vi "SetupAOTF.vi"() -> ()   [LabVIEW 2009]
uses:
  AOTFSettings.ctt
panel:
  in  "AOTF Setting":T1={"Laser 1 Output Channel"="5", "AOTF  1 Output Voltage"=5.0, "Laser 2 Output Channel"="6", "AOTF  2 Output Voltage"=5.0, "Laser 3 Output Channel"="1", "AOTF  3 Output Voltage"=0.0, "Pixel per Cycle"=3, "Time per Cycle  / ms"=0.1, "Laser 4 Output Channel"="1", "AOTF  4 Output Voltage"=0.0} {"AOTF  4 Output Voltage" format="%.2f"; "Time per Cycle  / ms" format="%#.3f"; "AOTF  3 Output Voltage" min=0.0 max=10.0 format="%.2f"; "AOTF  2 Output Voltage" min=0.0 max=10.0 format="%.2f"; "AOTF  1 Output Voltage" min=0.0 max=10.0 format="%.2f"}
  in  "Analog Setup":bool
  in  "OK Button":bool
  in  "Cancel Button":bool
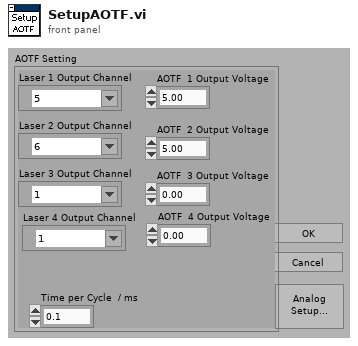
[diagram p1: front panel]
types:
  T1 = typedef "AOTFSettings.ctt" = cluster{"Laser 1 Output Channel":tag, "AOTF  1 Output Voltage":dbl, "Laser 2 Output Channel":tag, "AOTF  2 Output Voltage":dbl, "Laser 3 Output Channel":tag, "AOTF  3 Output Voltage":dbl, "Pixel per Cycle":u16, "Time per Cycle  / ms":dbl, "Laser 4 Output Channel":tag, "AOTF  4 Output Voltage":dbl}
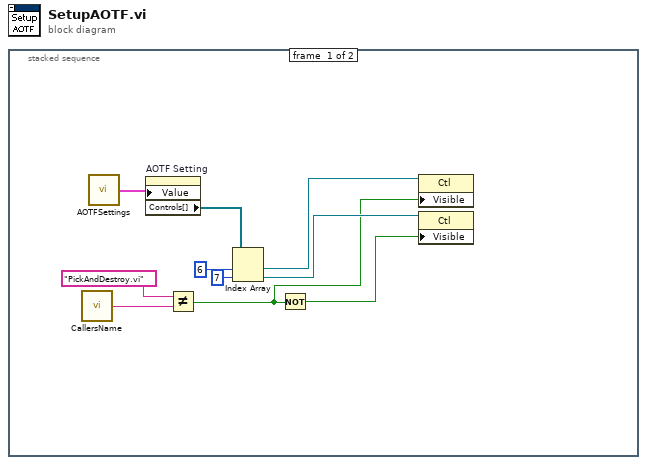
[diagram p0: block diagram]
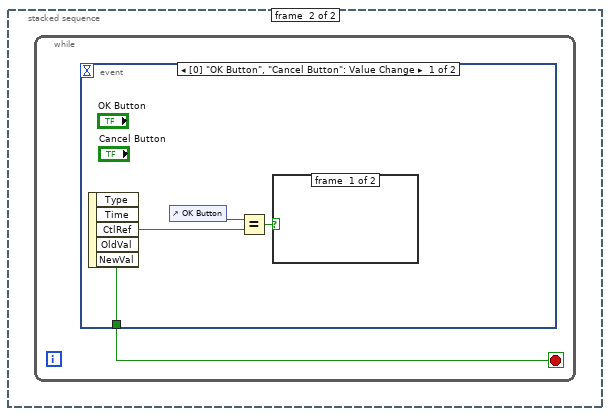
[diagram p2: hidden frame]
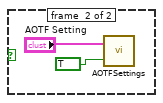
[diagram p3: hidden frame]
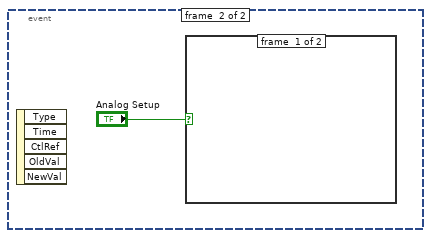
[diagram p4: hidden frame]
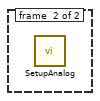
[diagram p5: hidden frame]
diagram:
  n1 = stacked-sequence {
    frame #0 {
      n2 = call "CallersName.vi"() -> ("Callers Name out"=w10:string)  [unwired: 2 in]
      n3 = call "AOTFSettings.vi"() -> ("AOTF Setting (Output)"=w8:T1)  [unwired: 2 in]
      n4 = property on="AOTF Setting" class="Cluster (strikt)"("Value"=w8) -> ("Controls[]"=w7:refnum<vi>[])  [unwired: 2 in, 2 out]
      n5 = Not Equal?(x="PickAndDestroy.vi", y=w10) -> (x != y?=w1:bool)
      n6 = Index Array(array=w7, index #1=6 ("index"), index #2=7 ("index")) -> (element #1=w6:refnum<vi>, element #2=w5:refnum<vi>)
      n7 = Not(x=w1) -> (.not. x?=w4:bool)
      n8 = property class="Ctl"(reference=w6, "Visible"=w1) -> ()  [unwired: 1 in, 2 out]
      n9 = property class="Ctl"(reference=w5, "Visible"=w4) -> ()  [unwired: 1 in, 2 out]
    }
    frame #1 {
      n10 = while {
        stop <- w11 stop-if-true
        n11 = event shown="[0] \"OK Button\", \"Cancel Button\": Value Change" {
          selector: _ -> [_ _]
          dyn-events: _ -> [_ _]
          timeout: _ -> [_ _]
          tunnel: [w14 _] -> w11
          event #0 {
            n12 = event-data() -> ("CtlRef"=w15:refnum<vi>, "NewVal"=w14:bool)  [unwired: 1 in, 3 out]
            n13 = control-ref of="OK Button"() -> (w13:refnum<vi>)
            n14 = Equal?(x=w13, y=w15) -> (x = y?=w12:bool)
            n15 = case shown="True" w12 {
              frame #0 {
              }
              frame #1 {
                n16 = call "AOTFSettings.vi"("Get/Set"=TRUE, "AOTF Setting (Input)"="AOTF Setting") -> ()  [unwired: 1 out]
              }
            }
          }
          event #1 {
            n17 = event-data() -> ()  [unwired: 1 in, 5 out]
            n18 = case shown="True" "Analog Setup" {
              frame #0 {
              }
              frame #1 {
                n19 = call "SetupAnalog.vi"() -> ()  [unwired: 1 in]
              }
            }
          }
        }
      }
    }
  }
